vi "VI Tree.vi"   [LabVIEW 2015, in "Rohde&Schwarz CMXP NR FR2 Measurement.lvlib"]
doc: "This is the instrument driver for the Rohde&Schwarz CMXP NR FR2 Measurement. \n\nThe VI Tree displays all the user-callable VIs of the instrument driver in an organized table.\n\nFor detailed driver information including modification history, refer to the <B>rscmxpnrfr2m.chm </B>file."
uses:
  <instrlib>/Rohde&Schwarz CMXP NR FR2 Measurement/Rohde&Schwarz CMXP NR FR2 Measurement.lvlib
panel:
  # "rsCmxpNrFr2M"
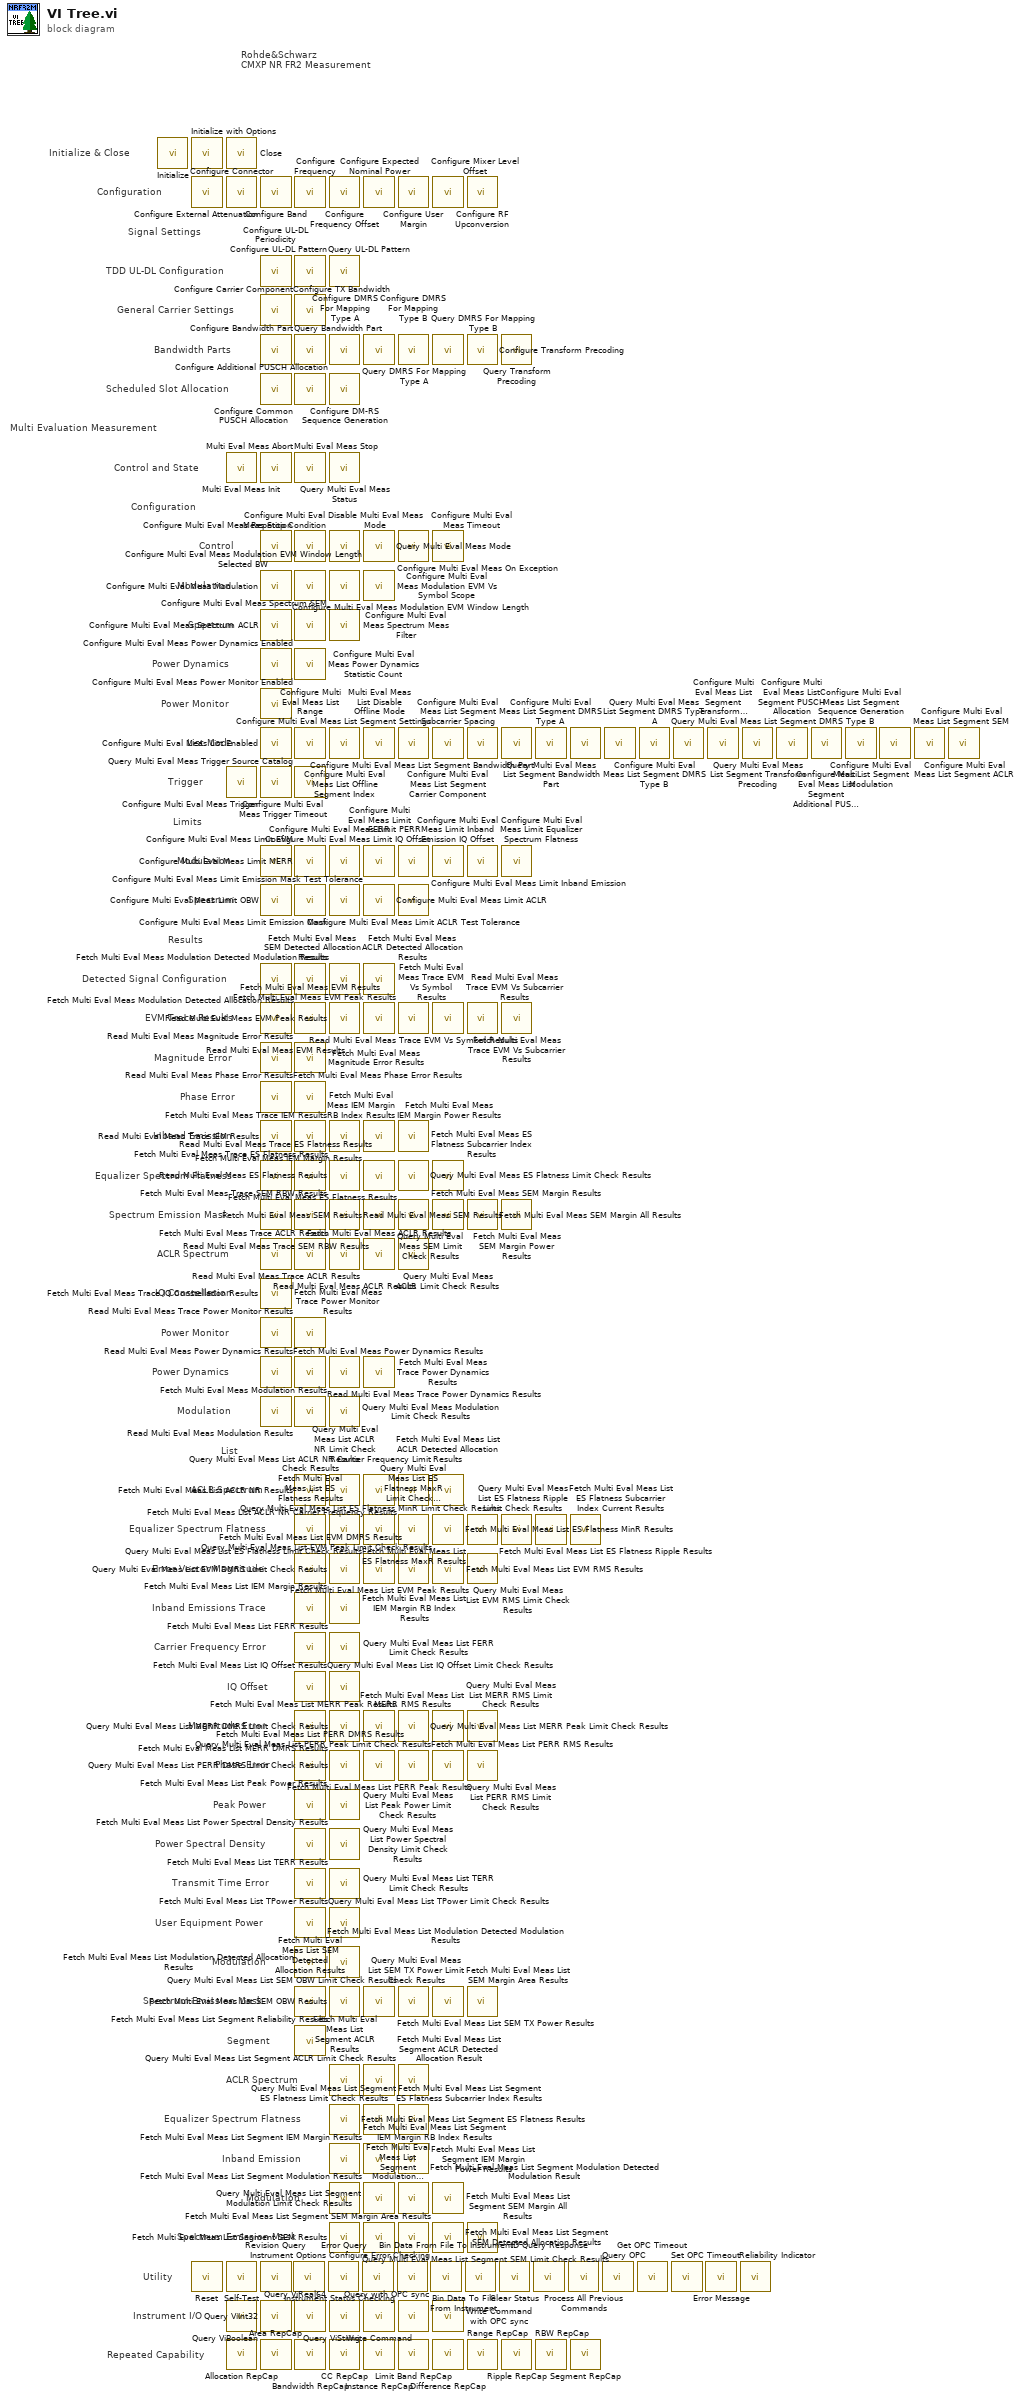
[diagram p0: block diagram]
diagram:
  # "Repeated Capability"
  # "Rohde&Schwarz \nCMXP NR FR2 Measurement"
  # "Instrument I/O"
  # "Utility"
  # "Spectrum Emission Mask"
  # "Modulation"
  # "Inband Emission"
  # "Equalizer Spectrum Flatness"
  # "ACLR Spectrum"
  # "Segment"
  # "Spectrum Emission Mask"
  # "Modulation"
  # "User Equipment Power"
  # "Transmit Time Error"
  # "Power Spectral Density"
  # "Peak Power"
  # "Phase Error"
  # "Magnitude Error"
  # "IQ Offset"
  # "Carrier Frequency Error"
  # "Inband Emissions Trace"
  # "Error Vector Magnitude"
  # "Equalizer Spectrum Flatness"
  # "ACLR Spectrum"
  # "List"
  # "Modulation"
  # "Power Dynamics"
  # "Power Monitor"
  # "IQ Constellation"
  # "ACLR Spectrum"
  # "Spectrum Emission Mask"
  # "Equalizer Spectrum Flatness"
  # "Inband Emission"
  # "Phase Error"
  # "Magnitude Error"
  # "EVM Trace Results"
  # "Detected Signal Configuration"
  # "Results"
  # "Control and State"
  # "Spectrum"
  # "Modulation"
  # "Limits"
  # "Trigger"
  # "List Mode"
  # "Power Monitor"
  # "Power Dynamics"
  # "Spectrum"
  # "Modulation"
  # "Control"
  # "Configuration"
  # "Multi Evaluation Measurement"
  # "Scheduled Slot Allocation"
  # "Bandwidth Parts"
  # "General Carrier Settings"
  # "TDD UL-DL Configuration"
  # "Signal Settings"
  # "Configuration"
  # "Initialize & Close"
  n1 = call <instrlib>:"Initialize.vi"() -> ()  [unwired: 10 in, 2 out]
  n2 = call <instrlib>:"Initialize with Options.vi"() -> ()  [unwired: 10 in, 2 out]
  n3 = call <instrlib>:"Configure Connector.vi"() -> ()  [unwired: 10 in, 2 out]
  n4 = call <instrlib>:"Reset.vi"() -> ()  [unwired: 10 in, 2 out]
  n5 = call <instrlib>:"Close.vi"() -> ()  [unwired: 11 in, 1 out]
  n6 = call <instrlib>:"Configure External Attenuation.vi"() -> ()  [unwired: 10 in, 2 out]
  n7 = call <instrlib>:"Multi Eval Meas Init.vi"() -> ()  [unwired: 10 in, 2 out]
  n8 = call <instrlib>:"Configure Multi Eval Meas Trigger.vi"() -> ()  [unwired: 10 in, 2 out]
  n9 = call <instrlib>:"Self-Test.vi"() -> ()  [unwired: 8 in, 4 out]
  n10 = call <instrlib>:"Query ViBoolean.vi"() -> ()  [unwired: 9 in, 3 out]
  n11 = call <instrlib>:"Allocation RepCap.vi"() -> ()  [unwired: 2 in, 2 out]
  n12 = call <instrlib>:"Configure Band.vi"() -> ()  [unwired: 10 in, 2 out]
  n13 = call <instrlib>:"Configure UL-DL Periodicity.vi"() -> ()  [unwired: 10 in, 2 out]
  n14 = call <instrlib>:"Configure Carrier Component.vi"() -> ()  [unwired: 10 in, 2 out]
  n15 = call <instrlib>:"Configure Bandwidth Part.vi"() -> ()  [unwired: 14 in, 2 out]
  n16 = call <instrlib>:"Configure Common PUSCH Allocation.vi"() -> ()  [unwired: 14 in, 2 out]
  n17 = call <instrlib>:"Multi Eval Meas Abort.vi"() -> ()  [unwired: 10 in, 2 out]
  n18 = call <instrlib>:"Configure Multi Eval Meas Repetition.vi"() -> ()  [unwired: 10 in, 2 out]
  n19 = call <instrlib>:"Configure Multi Eval Meas Modulation.vi"() -> ()  [unwired: 10 in, 2 out]
  n20 = call <instrlib>:"Configure Multi Eval Meas Spectrum ACLR.vi"() -> ()  [unwired: 10 in, 2 out]
  n21 = call <instrlib>:"Configure Multi Eval Meas Power Dynamics Enabled.vi"() -> ()  [unwired: 10 in, 2 out]
  n22 = call <instrlib>:"Configure Multi Eval Meas Power Monitor Enabled.vi"() -> ()  [unwired: 10 in, 2 out]
  n23 = call <instrlib>:"Configure Multi Eval Meas List Enabled.vi"() -> ()  [unwired: 10 in, 2 out]
  n24 = call <instrlib>:"Query Multi Eval Meas Trigger Source Catalog.vi"() -> ()  [unwired: 9 in, 3 out]
  n25 = call <instrlib>:"Configure Multi Eval Meas Limit EVM.vi"() -> ()  [unwired: 10 in, 2 out]
  n26 = call <instrlib>:"Configure Multi Eval Meas Limit OBW.vi"() -> ()  [unwired: 10 in, 2 out]
  n27 = call <instrlib>:"Fetch Multi Eval Meas Modulation Detected Allocation Results.vi"() -> ()  [unwired: 8 in, 4 out]
  n28 = call <instrlib>:"Read Multi Eval Meas EVM Results.vi"() -> ()  [unwired: 8 in, 4 out]
  n29 = call <instrlib>:"Read Multi Eval Meas Magnitude Error Results.vi"() -> ()  [unwired: 8 in, 4 out]
  n30 = call <instrlib>:"Read Multi Eval Meas Phase Error Results.vi"() -> ()  [unwired: 8 in, 4 out]
  n31 = call <instrlib>:"Read Multi Eval Meas Trace IEM Results.vi"() -> ()  [unwired: 8 in, 4 out]
  n32 = call <instrlib>:"Read Multi Eval Meas Trace ES Flatness Results.vi"() -> ()  [unwired: 8 in, 4 out]
  n33 = call <instrlib>:"Read Multi Eval Meas Trace SEM RBW Results.vi"() -> ()  [unwired: 8 in, 4 out]
  n34 = call <instrlib>:"Read Multi Eval Meas Trace ACLR Results.vi"() -> ()  [unwired: 8 in, 4 out]
  n35 = call <instrlib>:"Fetch Multi Eval Meas Trace IQ Constellation Results.vi"() -> ()  [unwired: 8 in, 4 out]
  n36 = call <instrlib>:"Read Multi Eval Meas Trace Power Monitor Results.vi"() -> ()  [unwired: 8 in, 4 out]
  n37 = call <instrlib>:"Read Multi Eval Meas Power Dynamics Results.vi"() -> ()  [unwired: 7 in, 5 out]
  n38 = call <instrlib>:"Read Multi Eval Meas Modulation Results.vi"() -> ()  [unwired: 8 in, 4 out]
  n39 = call <instrlib>:"Revision Query.vi"() -> ()  [unwired: 7 in, 5 out]
  n40 = call <instrlib>:"Query ViInt32.vi"() -> ()  [unwired: 9 in, 3 out]
  n41 = call <instrlib>:"Area RepCap.vi"() -> ()  [unwired: 2 in, 2 out]
  n42 = call <instrlib>:"Instrument Options.vi"() -> ()  [unwired: 9 in, 3 out]
  n43 = call <instrlib>:"Configure Frequency.vi"() -> ()  [unwired: 10 in, 2 out]
  n44 = call <instrlib>:"Configure UL-DL Pattern.vi"() -> ()  [unwired: 10 in, 2 out]
  n45 = call <instrlib>:"Configure TX Bandwidth.vi"() -> ()  [unwired: 10 in, 2 out]
  n46 = call <instrlib>:"Query Bandwidth Part.vi"() -> ()  [unwired: 6 in, 6 out]
  n47 = call <instrlib>:"Configure Additional PUSCH Allocation.vi"() -> ()  [unwired: 14 in, 2 out]
  n48 = call <instrlib>:"Multi Eval Meas Stop.vi"() -> ()  [unwired: 10 in, 2 out]
  n49 = call <instrlib>:"Configure Multi Eval Meas Stop Condition.vi"() -> ()  [unwired: 10 in, 2 out]
  n50 = call <instrlib>:"Configure Multi Eval Meas Modulation EVM Window Length.vi"() -> ()  [unwired: 10 in, 2 out]
  n51 = call <instrlib>:"Configure Multi Eval Meas Spectrum SEM.vi"() -> ()  [unwired: 10 in, 2 out]
  n52 = call <instrlib>:"Configure Multi Eval Meas Power Dynamics Statistic Count.vi"() -> ()  [unwired: 10 in, 2 out]
  n53 = call <instrlib>:"Configure Multi Eval Meas List Range.vi"() -> ()  [unwired: 10 in, 2 out]
  n54 = call <instrlib>:"Configure Multi Eval Meas Trigger Timeout.vi"() -> ()  [unwired: 10 in, 2 out]
  n55 = call <instrlib>:"Configure Multi Eval Meas Limit MERR.vi"() -> ()  [unwired: 10 in, 2 out]
  n56 = call <instrlib>:"Configure Multi Eval Meas Limit Emission Mask.vi"() -> ()  [unwired: 14 in, 2 out]
  n57 = call <instrlib>:"Fetch Multi Eval Meas Modulation Detected Modulation Results.vi"() -> ()  [unwired: 8 in, 4 out]
  n58 = call <instrlib>:"Fetch Multi Eval Meas EVM Results.vi"() -> ()  [unwired: 8 in, 4 out]
  n59 = call <instrlib>:"Fetch Multi Eval Meas Magnitude Error Results.vi"() -> ()  [unwired: 8 in, 4 out]
  n60 = call <instrlib>:"Fetch Multi Eval Meas Phase Error Results.vi"() -> ()  [unwired: 8 in, 4 out]
  n61 = call <instrlib>:"Fetch Multi Eval Meas Trace IEM Results.vi"() -> ()  [unwired: 8 in, 4 out]
  n62 = call <instrlib>:"Fetch Multi Eval Meas Trace ES Flatness Results.vi"() -> ()  [unwired: 8 in, 4 out]
  n63 = call <instrlib>:"Fetch Multi Eval Meas Trace SEM RBW Results.vi"() -> ()  [unwired: 8 in, 4 out]
  n64 = call <instrlib>:"Fetch Multi Eval Meas Trace ACLR Results.vi"() -> ()  [unwired: 8 in, 4 out]
  n65 = call <instrlib>:"Fetch Multi Eval Meas Trace Power Monitor Results.vi"() -> ()  [unwired: 8 in, 4 out]
  n66 = call <instrlib>:"Fetch Multi Eval Meas Power Dynamics Results.vi"() -> ()  [unwired: 7 in, 5 out]
  n67 = call <instrlib>:"Fetch Multi Eval Meas Modulation Results.vi"() -> ()  [unwired: 8 in, 4 out]
  n68 = call <instrlib>:"Fetch Multi Eval Meas List ACLR NR Results.vi"() -> ()  [unwired: 8 in, 4 out]
  n69 = call <instrlib>:"Fetch Multi Eval Meas List ES Flatness Results.vi"() -> ()  [unwired: 8 in, 4 out]
  n70 = call <instrlib>:"Fetch Multi Eval Meas List EVM DMRS Results.vi"() -> ()  [unwired: 8 in, 4 out]
  n71 = call <instrlib>:"Fetch Multi Eval Meas List IEM Margin Results.vi"() -> ()  [unwired: 8 in, 4 out]
  n72 = call <instrlib>:"Fetch Multi Eval Meas List FERR Results.vi"() -> ()  [unwired: 8 in, 4 out]
  n73 = call <instrlib>:"Fetch Multi Eval Meas List IQ Offset Results.vi"() -> ()  [unwired: 8 in, 4 out]
  n74 = call <instrlib>:"Fetch Multi Eval Meas List MERR DMRS Results.vi"() -> ()  [unwired: 8 in, 4 out]
  n75 = call <instrlib>:"Fetch Multi Eval Meas List PERR DMRS Results.vi"() -> ()  [unwired: 8 in, 4 out]
  n76 = call <instrlib>:"Fetch Multi Eval Meas List Peak Power Results.vi"() -> ()  [unwired: 8 in, 4 out]
  n77 = call <instrlib>:"Fetch Multi Eval Meas List Power Spectral Density Results.vi"() -> ()  [unwired: 8 in, 4 out]
  n78 = call <instrlib>:"Fetch Multi Eval Meas List TERR Results.vi"() -> ()  [unwired: 8 in, 4 out]
  n79 = call <instrlib>:"Fetch Multi Eval Meas List TPower Results.vi"() -> ()  [unwired: 8 in, 4 out]
  n80 = call <instrlib>:"Fetch Multi Eval Meas List Modulation Detected Allocation Results.vi"() -> ()  [unwired: 8 in, 4 out]
  n81 = call <instrlib>:"Fetch Multi Eval Meas List SEM Detected Allocation Results.vi"() -> ()  [unwired: 8 in, 4 out]
  n82 = call <instrlib>:"Fetch Multi Eval Meas List Segment Reliability Results.vi"() -> ()  [unwired: 8 in, 4 out]
  n83 = call <instrlib>:"Query ViReal64.vi"() -> ()  [unwired: 9 in, 3 out]
  n84 = call <instrlib>:"Bandwidth RepCap.vi"() -> ()  [unwired: 2 in, 2 out]
  n85 = call <instrlib>:"Error Query.vi"() -> ()  [unwired: 8 in, 4 out]
  n86 = call <instrlib>:"Configure Frequency Offset.vi"() -> ()  [unwired: 10 in, 2 out]
  n87 = call <instrlib>:"Query UL-DL Pattern.vi"() -> ()  [unwired: 6 in, 6 out]
  n88 = call <instrlib>:"Configure DMRS For Mapping Type A.vi"() -> ()  [unwired: 10 in, 2 out]
  n89 = call <instrlib>:"Configure DM-RS Sequence Generation.vi"() -> ()  [unwired: 10 in, 2 out]
  n90 = call <instrlib>:"Query Multi Eval Meas Status.vi"() -> ()  [unwired: 7 in, 5 out]
  n91 = call <instrlib>:"Disable Multi Eval Meas Mode.vi"() -> ()  [unwired: 10 in, 2 out]
  n92 = call <instrlib>:"Configure Multi Eval Meas Modulation EVM Window Length Selected BW.vi"() -> ()  [unwired: 10 in, 2 out]
  n93 = call <instrlib>:"Configure Multi Eval Meas Spectrum Meas Filter.vi"() -> ()  [unwired: 10 in, 2 out]
  n94 = call <instrlib>:"Configure Multi Eval Meas List Offline Segment Index.vi"() -> ()  [unwired: 10 in, 2 out]
  n95 = call <instrlib>:"Configure Multi Eval Meas Limit PERR.vi"() -> ()  [unwired: 10 in, 2 out]
  n96 = call <instrlib>:"Configure Multi Eval Meas Limit Emission Mask Test Tolerance.vi"() -> ()  [unwired: 10 in, 2 out]
  n97 = call <instrlib>:"Fetch Multi Eval Meas SEM Detected Allocation Results.vi"() -> ()  [unwired: 8 in, 4 out]
  n98 = call <instrlib>:"Read Multi Eval Meas EVM Peak Results.vi"() -> ()  [unwired: 8 in, 4 out]
  n99 = call <instrlib>:"Fetch Multi Eval Meas IEM Margin Results.vi"() -> ()  [unwired: 8 in, 4 out]
  n100 = call <instrlib>:"Read Multi Eval Meas ES Flatness Results.vi"() -> ()  [unwired: 8 in, 4 out]
  n101 = call <instrlib>:"Read Multi Eval Meas SEM Results.vi"() -> ()  [unwired: 8 in, 4 out]
  n102 = call <instrlib>:"Read Multi Eval Meas ACLR Results.vi"() -> ()  [unwired: 8 in, 4 out]
  n103 = call <instrlib>:"Read Multi Eval Meas Trace Power Dynamics Results.vi"() -> ()  [unwired: 8 in, 4 out]
  n104 = call <instrlib>:"Query Multi Eval Meas Modulation Limit Check Results.vi"() -> ()  [unwired: 8 in, 4 out]
  n105 = call <instrlib>:"Query Multi Eval Meas List ACLR NR Limit Check Results.vi"() -> ()  [unwired: 8 in, 4 out]
  n106 = call <instrlib>:"Query Multi Eval Meas List ES Flatness Limit Check Results.vi"() -> ()  [unwired: 8 in, 4 out]
  n107 = call <instrlib>:"Query Multi Eval Meas List EVM DMRS Limit Check Results.vi"() -> ()  [unwired: 8 in, 4 out]
  n108 = call <instrlib>:"Fetch Multi Eval Meas List IEM Margin RB Index Results.vi"() -> ()  [unwired: 8 in, 4 out]
  n109 = call <instrlib>:"Query Multi Eval Meas List FERR Limit Check Results.vi"() -> ()  [unwired: 8 in, 4 out]
  n110 = call <instrlib>:"Query Multi Eval Meas List IQ Offset Limit Check Results.vi"() -> ()  [unwired: 8 in, 4 out]
  n111 = call <instrlib>:"Query Multi Eval Meas List MERR DMRS Limit Check Results.vi"() -> ()  [unwired: 8 in, 4 out]
  n112 = call <instrlib>:"Query Multi Eval Meas List PERR DMRS Limit Check Results.vi"() -> ()  [unwired: 8 in, 4 out]
  n113 = call <instrlib>:"Query Multi Eval Meas List Peak Power Limit Check Results.vi"() -> ()  [unwired: 8 in, 4 out]
  n114 = call <instrlib>:"Query Multi Eval Meas List Power Spectral Density Limit Check Results.vi"() -> ()  [unwired: 8 in, 4 out]
  n115 = call <instrlib>:"Query Multi Eval Meas List TERR Limit Check Results.vi"() -> ()  [unwired: 8 in, 4 out]
  n116 = call <instrlib>:"Query Multi Eval Meas List TPower Limit Check Results.vi"() -> ()  [unwired: 8 in, 4 out]
  n117 = call <instrlib>:"Fetch Multi Eval Meas List Modulation Detected Modulation Results.vi"() -> ()  [unwired: 8 in, 4 out]
  n118 = call <instrlib>:"Fetch Multi Eval Meas List SEM OBW Results.vi"() -> ()  [unwired: 8 in, 4 out]
  n119 = call <instrlib>:"Fetch Multi Eval Meas List Segment ACLR Results.vi"() -> ()  [unwired: 6 in, 6 out]
  n120 = call <instrlib>:"Fetch Multi Eval Meas List Segment ES Flatness Results.vi"() -> ()  [unwired: 6 in, 6 out]
  n121 = call <instrlib>:"Fetch Multi Eval Meas List Segment IEM Margin Results.vi"() -> ()  [unwired: 6 in, 6 out]
  n122 = call <instrlib>:"Fetch Multi Eval Meas List Segment Modulation Results.vi"() -> ()  [unwired: 6 in, 6 out]
  n123 = call <instrlib>:"Fetch Multi Eval Meas List Segment SEM Results.vi"() -> ()  [unwired: 6 in, 6 out]
  n124 = call <instrlib>:"Query ViString.vi"() -> ()  [unwired: 9 in, 3 out]
  n125 = call <instrlib>:"CC RepCap.vi"() -> ()  [unwired: 2 in, 2 out]
  n126 = call <instrlib>:"Instrument Status Checking.vi"() -> ()  [unwired: 10 in, 2 out]
  n127 = call <instrlib>:"Configure Expected Nominal Power.vi"() -> ()  [unwired: 10 in, 2 out]
  n128 = call <instrlib>:"Query DMRS For Mapping Type A.vi"() -> ()  [unwired: 7 in, 5 out]
  n129 = call <instrlib>:"Query Multi Eval Meas Mode.vi"() -> ()  [unwired: 9 in, 3 out]
  n130 = call <instrlib>:"Configure Multi Eval Meas Modulation EVM Vs Symbol Scope.vi"() -> ()  [unwired: 10 in, 2 out]
  n131 = call <instrlib>:"Multi Eval Meas List Disable Offline Mode.vi"() -> ()  [unwired: 10 in, 2 out]
  n132 = call <instrlib>:"Configure Multi Eval Meas Limit FERR.vi"() -> ()  [unwired: 10 in, 2 out]
  n133 = call <instrlib>:"Configure Multi Eval Meas Limit ACLR.vi"() -> ()  [unwired: 14 in, 2 out]
  n134 = call <instrlib>:"Fetch Multi Eval Meas ACLR Detected Allocation Results.vi"() -> ()  [unwired: 8 in, 4 out]
  n135 = call <instrlib>:"Fetch Multi Eval Meas EVM Peak Results.vi"() -> ()  [unwired: 8 in, 4 out]
  n136 = call <instrlib>:"Fetch Multi Eval Meas IEM Margin RB Index Results.vi"() -> ()  [unwired: 8 in, 4 out]
  n137 = call <instrlib>:"Fetch Multi Eval Meas ES Flatness Results.vi"() -> ()  [unwired: 8 in, 4 out]
  n138 = call <instrlib>:"Fetch Multi Eval Meas SEM Results.vi"() -> ()  [unwired: 8 in, 4 out]
  n139 = call <instrlib>:"Fetch Multi Eval Meas ACLR Results.vi"() -> ()  [unwired: 8 in, 4 out]
  n140 = call <instrlib>:"Fetch Multi Eval Meas Trace Power Dynamics Results.vi"() -> ()  [unwired: 8 in, 4 out]
  n141 = call <instrlib>:"Fetch Multi Eval Meas List ACLR NR Carrier Frequency Results.vi"() -> ()  [unwired: 8 in, 4 out]
  n142 = call <instrlib>:"Fetch Multi Eval Meas List ES Flatness MaxR Results.vi"() -> ()  [unwired: 8 in, 4 out]
  n143 = call <instrlib>:"Fetch Multi Eval Meas List EVM Peak Results.vi"() -> ()  [unwired: 8 in, 4 out]
  n144 = call <instrlib>:"Fetch Multi Eval Meas List MERR Peak Results.vi"() -> ()  [unwired: 8 in, 4 out]
  n145 = call <instrlib>:"Fetch Multi Eval Meas List PERR Peak Results.vi"() -> ()  [unwired: 8 in, 4 out]
  n146 = call <instrlib>:"Query Multi Eval Meas List SEM OBW Limit Check Results.vi"() -> ()  [unwired: 8 in, 4 out]
  n147 = call <instrlib>:"Query Multi Eval Meas List Segment ACLR Limit Check Results.vi"() -> ()  [unwired: 6 in, 6 out]
  n148 = call <instrlib>:"Query Multi Eval Meas List Segment ES Flatness Limit Check Results.vi"() -> ()  [unwired: 6 in, 6 out]
  n149 = call <instrlib>:"Fetch Multi Eval Meas List Segment IEM Margin RB Index Results.vi"() -> ()  [unwired: 6 in, 6 out]
  n150 = call <instrlib>:"Query Multi Eval Meas List Segment Modulation Limit Check Results.vi"() -> ()  [unwired: 6 in, 6 out]
  n151 = call <instrlib>:"Query Multi Eval Meas List Segment SEM Limit Check Results.vi"() -> ()  [unwired: 6 in, 6 out]
  n152 = call <instrlib>:"Write Command.vi"() -> ()  [unwired: 10 in, 2 out]
  n153 = call <instrlib>:"Instance RepCap.vi"() -> ()  [unwired: 2 in, 2 out]
  n154 = call <instrlib>:"Configure Error Checking.vi"() -> ()  [unwired: 10 in, 2 out]
  n155 = call <instrlib>:"Configure User Margin.vi"() -> ()  [unwired: 10 in, 2 out]
  n156 = call <instrlib>:"Configure DMRS For Mapping Type B.vi"() -> ()  [unwired: 10 in, 2 out]
  n157 = call <instrlib>:"Configure Multi Eval Meas On Exception.vi"() -> ()  [unwired: 10 in, 2 out]
  n158 = call <instrlib>:"Configure Multi Eval Meas List Segment Settings.vi"() -> ()  [unwired: 14 in, 2 out]
  n159 = call <instrlib>:"Configure Multi Eval Meas Limit IQ Offset.vi"() -> ()  [unwired: 10 in, 2 out]
  n160 = call <instrlib>:"Configure Multi Eval Meas Limit ACLR Test Tolerance.vi"() -> ()  [unwired: 10 in, 2 out]
  n161 = call <instrlib>:"Read Multi Eval Meas Trace EVM Vs Symbol Results.vi"() -> ()  [unwired: 8 in, 4 out]
  n162 = call <instrlib>:"Fetch Multi Eval Meas IEM Margin Power Results.vi"() -> ()  [unwired: 8 in, 4 out]
  n163 = call <instrlib>:"Query Multi Eval Meas ES Flatness Limit Check Results.vi"() -> ()  [unwired: 8 in, 4 out]
  n164 = call <instrlib>:"Query Multi Eval Meas SEM Limit Check Results.vi"() -> ()  [unwired: 8 in, 4 out]
  n165 = call <instrlib>:"Query Multi Eval Meas ACLR Limit Check Results.vi"() -> ()  [unwired: 8 in, 4 out]
  n166 = call <instrlib>:"Query Multi Eval Meas List ACLR NR Carrier Frequency Limit Check Results.vi"() -> ()  [unwired: 8 in, 4 out]
  n167 = call <instrlib>:"Query Multi Eval Meas List ES Flatness MaxR Limit Check Results.vi"() -> ()  [unwired: 8 in, 4 out]
  n168 = call <instrlib>:"Query Multi Eval Meas List EVM Peak Limit Check Results.vi"() -> ()  [unwired: 8 in, 4 out]
  n169 = call <instrlib>:"Query Multi Eval Meas List MERR Peak Limit Check Results.vi"() -> ()  [unwired: 8 in, 4 out]
  n170 = call <instrlib>:"Query Multi Eval Meas List PERR Peak Limit Check Results.vi"() -> ()  [unwired: 8 in, 4 out]
  n171 = call <instrlib>:"Fetch Multi Eval Meas List SEM TX Power Results.vi"() -> ()  [unwired: 8 in, 4 out]
  n172 = call <instrlib>:"Fetch Multi Eval Meas List Segment ACLR Detected Allocation Result.vi"() -> ()  [unwired: 8 in, 4 out]
  n173 = call <instrlib>:"Fetch Multi Eval Meas List Segment ES Flatness Subcarrier Index Results.vi"() -> ()  [unwired: 6 in, 6 out]
  n174 = call <instrlib>:"Fetch Multi Eval Meas List Segment IEM Margin Power Results.vi"() -> ()  [unwired: 6 in, 6 out]
  n175 = call <instrlib>:"Fetch Multi Eval Meas List Segment Modulation Detected Allocation Result.vi"() -> ()  [unwired: 8 in, 4 out]
  n176 = call <instrlib>:"Fetch Multi Eval Meas List Segment SEM Margin Area Results.vi"() -> ()  [unwired: 6 in, 6 out]
  n177 = call <instrlib>:"Query with OPC sync.vi"() -> ()  [unwired: 9 in, 3 out]
  n178 = call <instrlib>:"Limit Band RepCap.vi"() -> ()  [unwired: 2 in, 2 out]
  n179 = call <instrlib>:"Bin Data From File To Instrument.vi"() -> ()  [unwired: 10 in, 2 out]
  n180 = call <instrlib>:"Configure Mixer Level Offset.vi"() -> ()  [unwired: 10 in, 2 out]
  n181 = call <instrlib>:"Query DMRS For Mapping Type B.vi"() -> ()  [unwired: 7 in, 5 out]
  n182 = call <instrlib>:"Configure Multi Eval Meas Timeout.vi"() -> ()  [unwired: 10 in, 2 out]
  n183 = call <instrlib>:"Configure Multi Eval Meas List Segment Carrier Component.vi"() -> ()  [unwired: 14 in, 2 out]
  n184 = call <instrlib>:"Configure Multi Eval Meas Limit Inband Emission.vi"() -> ()  [unwired: 14 in, 2 out]
  n185 = call <instrlib>:"Fetch Multi Eval Meas Trace EVM Vs Symbol Results.vi"() -> ()  [unwired: 8 in, 4 out]
  n186 = call <instrlib>:"Fetch Multi Eval Meas ES Flatness Subcarrier Index Results.vi"() -> ()  [unwired: 8 in, 4 out]
  n187 = call <instrlib>:"Fetch Multi Eval Meas SEM Margin Results.vi"() -> ()  [unwired: 7 in, 5 out]
  n188 = call <instrlib>:"Fetch Multi Eval Meas List ACLR Detected Allocation Results.vi"() -> ()  [unwired: 9 in, 3 out]
  n189 = call <instrlib>:"Fetch Multi Eval Meas List ES Flatness MinR Results.vi"() -> ()  [unwired: 8 in, 4 out]
  n190 = call <instrlib>:"Fetch Multi Eval Meas List EVM RMS Results.vi"() -> ()  [unwired: 8 in, 4 out]
  n191 = call <instrlib>:"Fetch Multi Eval Meas List MERR RMS Results.vi"() -> ()  [unwired: 8 in, 4 out]
  n192 = call <instrlib>:"Fetch Multi Eval Meas List PERR RMS Results.vi"() -> ()  [unwired: 8 in, 4 out]
  n193 = call <instrlib>:"Query Multi Eval Meas List SEM TX Power Limit Check Results.vi"() -> ()  [unwired: 8 in, 4 out]
  n194 = call <instrlib>:"Fetch Multi Eval Meas List Segment Modulation Detected Modulation Result.vi"() -> ()  [unwired: 8 in, 4 out]
  n195 = call <instrlib>:"Fetch Multi Eval Meas List Segment SEM Detected Allocation Results.vi"() -> ()  [unwired: 8 in, 4 out]
  n196 = call <instrlib>:"Write Command with OPC sync.vi"() -> ()  [unwired: 10 in, 2 out]
  n197 = call <instrlib>:"Difference RepCap.vi"() -> ()  [unwired: 2 in, 2 out]
  n198 = call <instrlib>:"Bin Data To File From Instrument.vi"() -> ()  [unwired: 10 in, 2 out]
  n199 = call <instrlib>:"Configure RF Upconversion.vi"() -> ()  [unwired: 10 in, 2 out]
  n200 = call <instrlib>:"Configure Transform Precoding.vi"() -> ()  [unwired: 10 in, 2 out]
  n201 = call <instrlib>:"Configure Multi Eval Meas List Segment Subcarrier Spacing.vi"() -> ()  [unwired: 10 in, 2 out]
  n202 = call <instrlib>:"Configure Multi Eval Meas Limit Inband Emission IQ Offset.vi"() -> ()  [unwired: 10 in, 2 out]
  n203 = call <instrlib>:"Read Multi Eval Meas Trace EVM Vs Subcarrier Results.vi"() -> ()  [unwired: 8 in, 4 out]
  n204 = call <instrlib>:"Fetch Multi Eval Meas SEM Margin All Results.vi"() -> ()  [unwired: 7 in, 5 out]
  n205 = call <instrlib>:"Query Multi Eval Meas List ES Flatness MinR Limit Check Results.vi"() -> ()  [unwired: 8 in, 4 out]
  n206 = call <instrlib>:"Query Multi Eval Meas List EVM RMS Limit Check Results.vi"() -> ()  [unwired: 8 in, 4 out]
  n207 = call <instrlib>:"Query Multi Eval Meas List MERR RMS Limit Check Results.vi"() -> ()  [unwired: 8 in, 4 out]
  n208 = call <instrlib>:"Query Multi Eval Meas List PERR RMS Limit Check Results.vi"() -> ()  [unwired: 8 in, 4 out]
  n209 = call <instrlib>:"Fetch Multi Eval Meas List SEM Margin Area Results.vi"() -> ()  [unwired: 9 in, 3 out]
  n210 = call <instrlib>:"Fetch Multi Eval Meas List Segment SEM Margin All Results.vi"() -> ()  [unwired: 6 in, 6 out]
  n211 = call <instrlib>:"Range RepCap.vi"() -> ()  [unwired: 2 in, 2 out]
  n212 = call <instrlib>:"Clear Status.vi"() -> ()  [unwired: 10 in, 2 out]
  n213 = call <instrlib>:"Query Transform Precoding.vi"() -> ()  [unwired: 9 in, 3 out]
  n214 = call <instrlib>:"Configure Multi Eval Meas List Segment Bandwidth Part.vi"() -> ()  [unwired: 14 in, 2 out]
  n215 = call <instrlib>:"Configure Multi Eval Meas Limit Equalizer Spectrum Flatness.vi"() -> ()  [unwired: 14 in, 2 out]
  n216 = call <instrlib>:"Fetch Multi Eval Meas Trace EVM Vs Subcarrier Results.vi"() -> ()  [unwired: 8 in, 4 out]
  n217 = call <instrlib>:"Fetch Multi Eval Meas SEM Margin Power Results.vi"() -> ()  [unwired: 7 in, 5 out]
  n218 = call <instrlib>:"Fetch Multi Eval Meas List ES Flatness Ripple Results.vi"() -> ()  [unwired: 8 in, 4 out]
  n219 = call <instrlib>:"Ripple RepCap.vi"() -> ()  [unwired: 2 in, 2 out]
  n220 = call <instrlib>:"ID Query Response.vi"() -> ()  [unwired: 9 in, 3 out]
  n221 = call <instrlib>:"Query Multi Eval Meas List Segment Bandwidth Part.vi"() -> ()  [unwired: 6 in, 6 out]
  n222 = call <instrlib>:"Query Multi Eval Meas List ES Flatness Ripple Limit Check Results.vi"() -> ()  [unwired: 8 in, 4 out]
  n223 = call <instrlib>:"RBW RepCap.vi"() -> ()  [unwired: 2 in, 2 out]
  n224 = call <instrlib>:"Process All Previous Commands.vi"() -> ()  [unwired: 10 in, 2 out]
  n225 = call <instrlib>:"Configure Multi Eval Meas List Segment DMRS Type A.vi"() -> ()  [unwired: 10 in, 2 out]
  n226 = call <instrlib>:"Fetch Multi Eval Meas List ES Flatness Subcarrier Index Current Results.vi"() -> ()  [unwired: 8 in, 4 out]
  n227 = call <instrlib>:"Segment RepCap.vi"() -> ()  [unwired: 2 in, 2 out]
  n228 = call <instrlib>:"Query OPC.vi"() -> ()  [unwired: 9 in, 3 out]
  n229 = call <instrlib>:"Query Multi Eval Meas List Segment DMRS Type A.vi"() -> ()  [unwired: 7 in, 5 out]
  n230 = call <instrlib>:"Get OPC Timeout.vi"() -> ()  [unwired: 9 in, 3 out]
  n231 = call <instrlib>:"Configure Multi Eval Meas List Segment DMRS Type B.vi"() -> ()  [unwired: 10 in, 2 out]
  n232 = call <instrlib>:"Set OPC Timeout.vi"() -> ()  [unwired: 10 in, 2 out]
  n233 = call <instrlib>:"Query Multi Eval Meas List Segment DMRS Type B.vi"() -> ()  [unwired: 7 in, 5 out]
  n234 = call <instrlib>:"Error Message.vi"() -> ()  [unwired: 7 in, 5 out]
  n235 = call <instrlib>:"Configure Multi Eval Meas List Segment Transform Precoding.vi"() -> ()  [unwired: 10 in, 2 out]
  n236 = call <instrlib>:"Reliability Indicator.vi"() -> ()  [unwired: 9 in, 3 out]
  n237 = call <instrlib>:"Query Multi Eval Meas List Segment Transform Precoding.vi"() -> ()  [unwired: 9 in, 3 out]
  n238 = call <instrlib>:"Configure Multi Eval Meas List Segment PUSCH Allocation.vi"() -> ()  [unwired: 14 in, 2 out]
  n239 = call <instrlib>:"Configure Multi Eval Meas List Segment Additional PUSCH Allocation.vi"() -> ()  [unwired: 14 in, 2 out]
  n240 = call <instrlib>:"Configure Multi Eval Meas List Segment Sequence Generation.vi"() -> ()  [unwired: 14 in, 2 out]
  n241 = call <instrlib>:"Configure Multi Eval Meas List Segment Modulation.vi"() -> ()  [unwired: 10 in, 2 out]
  n242 = call <instrlib>:"Configure Multi Eval Meas List Segment SEM.vi"() -> ()  [unwired: 10 in, 2 out]
  n243 = call <instrlib>:"Configure Multi Eval Meas List Segment ACLR.vi"() -> ()  [unwired: 10 in, 2 out]
